vi "Remove Section.vi"(8 "error in (no error)":errorcluster, 10 "Section":string, 11 "configuration file path":path) -> (0 "error out":errorcluster)   [LabVIEW 2015]
uses:
  <vilib>/regexp/Match Regular Expression.xnode
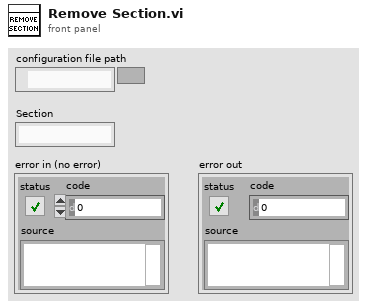
[diagram p1: front panel]
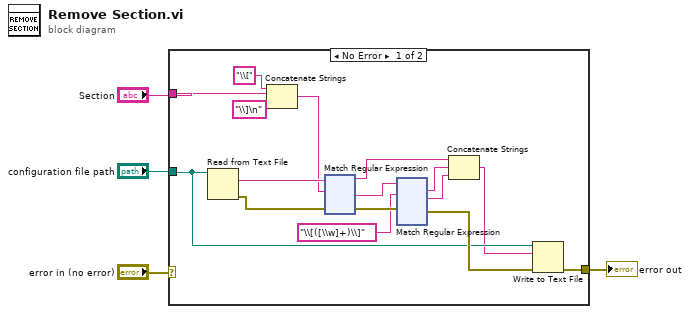
[diagram p0: block diagram]
diagram:
  n1 = case shown="No Error" "error in (no error)" {
    selector: "error in (no error)" -> [_ w245]
    tunnel: "Section" -> [w19 _]
    tunnel: [w5 w245] -> w2
    tunnel: "configuration file path" -> [w7 _]
    frame No Error {
      n2 = Read from Text File(file (use dialog)=w7) -> (text=w20:string, error out=w15:errorcluster)  [unwired: 3 in, 2 out]
      n3 = Concatenate Strings("\\[", w19, "\\]\n") -> (w16:string)
      n4 = xnode "Match Regular Expression"("input string"=w20, "regular expression"=w16, "error in"=w15) -> ("before match"=w10:string, "after match"=w13:string, "error out"=w14:errorcluster)  [unwired: 3 in, 2 out]
      n5 = xnode "Match Regular Expression"("input string"=w13, "regular expression"="\\[([\\w]+)\\]", "error in"=w14) -> ("whole match"=w9:string, "after match"=w11:string, "error out"=w8:errorcluster)  [unwired: 3 in, 3 out]
      n6 = Concatenate Strings(w10, w9, w11) -> (w6:string)
      n7 = Write to Text File(file (use dialog)=w7, text=w6, error in=w8) -> (error out=w5:errorcluster)  [unwired: 1 in, 2 out]
    }
    frame Error {
    }
  }
  "error out" <- w2
